vi "Build Dll.vi"(8 "error in":errorcluster, 11 "csproj Path in":path) -> (0 "error out":errorcluster, 3 "csproj Path out":path)   [LabVIEW 2026, in "NIVS_CDEW_MetaDataObj.lvclass"]
uses:
  NIVS_CDEW_MetaDataObj.lvclass
  NIVS_CDEW_MetaDataObj.lvclass/NIVS_CDEW_MetaDataObj.ctl
  Types/Errors.ctl
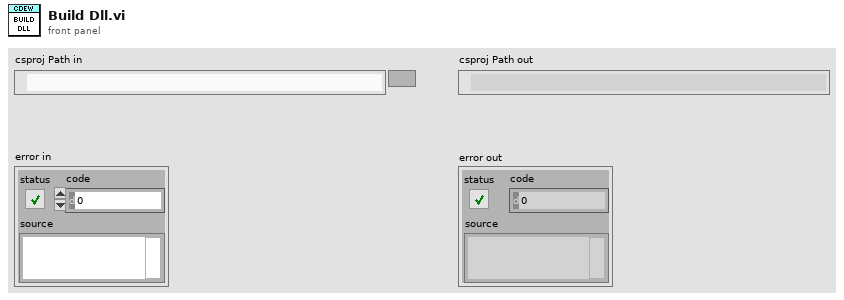
[diagram p1: front panel]
types:
  T1 = typedef "NIVS_CDEW_MetaDataObj.lvclass/Errors.ctl" = i32
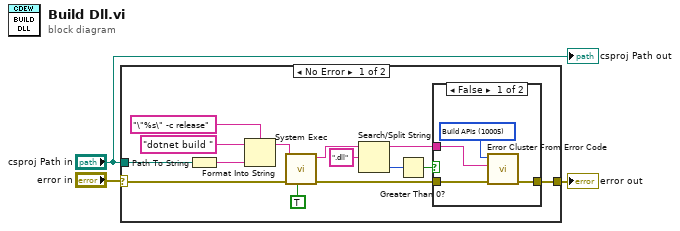
[diagram p0: block diagram]
diagram:
  n1 = case shown="No Error" "error in" {
    selector: "error in" -> [w14 w23]
    tunnel: [w5 w23] -> w2
    tunnel: "csproj Path in" -> [w12 _]
    frame No Error {
      n2 = Path To String(path=w12) -> (string=w16:string)
      n3 = Format Into String(format string="\"%s\" -c release", initial string="dotnet build ", w16) -> (resulting string=w15:string)  [unwired: 1 in, 1 out]
      n4 = call <vilib>:"System Exec.vi"("run minimized? (F)"=TRUE, "error in (no error)"=w14, "command line"=w15) -> ("error out"=w6:errorcluster, "standard output"=w10:string)  [unwired: 5 in, 2 out]
      n5 = Search/Split String(string=w10, search string/char (-)=".dll") -> (substring before match=w4:string, offset of match=w8:i32)  [unwired: 1 in, 1 out]
      n6 = Greater Than 0?(x=w8) -> (x > 0?=w7:bool)
      n7 = case shown="False" w7 {
        tunnel: w6 -> [w21 w22]
        tunnel: [w20 w22] -> w5
        tunnel: w4 -> [w18 _]
        frame False {
          w19 = T1 10005 items=["Invalid XML File"=10001, "Missing File/Folder"=10002, "Duplicate CD in Root"=10003, "API Auto Gen"=10004, "Build APIs"=10005, "Clusters Auto Gen"=10006, "Create LV Projects"=10007] ("Errors")
          n8 = call <vilib>:"Error Cluster From Error Code.vi"("error in (no error)"=w21, "error message (\"\")"=w18, "error code (0)"=w19) -> ("error out"=w20:errorcluster)  [unwired: 6 in]
        }
        frame True {
        }
      }
    }
    frame Error {
    }
  }
  "error out" <- w2
  "csproj Path out" <- "csproj Path in"
